vi "String3.vi"() -> ()   [LabVIEW 2020]
panel:
  in  "width (-)":i16
  out "x+1":i32
  out "decimal integer string":string
  in  "number":i32
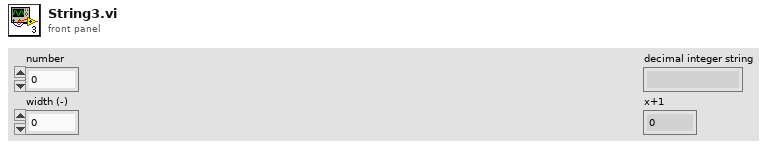
[diagram p1: front panel]
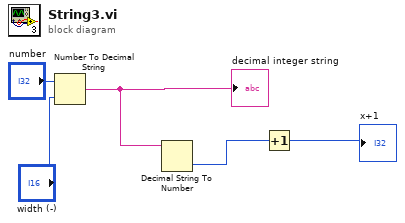
[diagram p0: block diagram]
diagram:
  n1 = Number To Decimal String(number="number", width (-)="width (-)") -> (decimal integer string=w4:string)
  "decimal integer string" <- w4
  n2 = Decimal String To Number(string=w4) -> (number=w3:i32)  [unwired: 2 in, 1 out]
  n3 = Increment(x=w3) -> (x+1=→"x+1":i32)
